vi "PathPlanner_Trajectory_Sample.vi"(9 "Time":dbl, 11 "PathPlannerTrajectory":T6 {"States"."HolonomicRotation"."SIN" format="%13.4f"; "States"."HolonomicRotation"."COS" format="%13.4f"; "States"."HolonomicRotation"."VALUE" format="%13.4f"; "States"."AngularVelocity"."SIN" format="%13.4f"; "States"."AngularVelocity"."COS" format="%13.4f"; "States"."AngularVelocity"."VALUE" format="%13.4f"; "States"."TrajectoryState"."POSE"."ROTATION"."SIN" format="%13.4f"; "States"."TrajectoryState"."POSE"."ROTATION"."COS" format="%13.4f"; "States"."TrajectoryState"."POSE"."ROTATION"."VALUE" format="%13.4f"; "States"."TrajectoryState"."POSE"."TRANSLATION"."Y" format="%14.3f"; "States"."TrajectoryState"."POSE"."TRANSLATION"."X" format="%14.3f"; "States"."AngularAcceleration"."SIN" format="%13.4f"; "States"."AngularAcceleration"."COS" format="%13.4f"; "States"."AngularAcceleration"."VALUE" format="%13.4f"}) -> (3 "PathPlannerState":T1={"AngularAcceleration"={"VALUE"=0.0, "COS"=1.0, "SIN"=0.0}, "PositionMeters"=0.0, "TrajectoryState"={"TimeSeconds"=0.0, "Velocity"=0.0, "Acceleration"=0.0, "POSE"={"TRANSLATION"={"X"=0.0, "Y"=0.0}, "ROTATION"={"VALUE"=0.0, "COS"=1.0, "SIN"=0.0}}, "Curvature"=0.0}, "AngularVelocity"={"VALUE"=0.0, "COS"=1.0, "SIN"=0.0}, "HolonomicRotation"={"VALUE"=0.0, "COS"=1.0, "SIN"=0.0}, "CurveRadius"=0.0, "DeltaPos"=0.0} {"HolonomicRotation"."SIN" format="%13.4f"; "HolonomicRotation"."COS" format="%13.4f"; "HolonomicRotation"."VALUE" format="%13.4f"; "AngularVelocity"."SIN" format="%13.4f"; "AngularVelocity"."COS" format="%13.4f"; "AngularVelocity"."VALUE" format="%13.4f"; "TrajectoryState"."POSE"."ROTATION"."SIN" format="%13.4f"; "TrajectoryState"."POSE"."ROTATION"."COS" format="%13.4f"; "TrajectoryState"."POSE"."ROTATION"."VALUE" format="%13.4f"; "TrajectoryState"."POSE"."TRANSLATION"."Y" format="%14.3f"; "TrajectoryState"."POSE"."TRANSLATION"."X" format="%14.3f"; "AngularAcceleration"."SIN" format="%13.4f"; "AngularAcceleration"."COS" format="%13.4f"; "AngularAcceleration"."VALUE" format="%13.4f"})   [LabVIEW 2019, in "PathPlanner.lvlib"]
doc: "Sample the path at a point in time\n\nInputs:\n - time -- The time to sample\n\nOutputs:\n - PathPlannerState -- The state at the given point in time"
uses:
  PathPlanner.lvlib
  PathPlannerTrajectory.ctl
  PathPlannerState.ctl
  <vilib>/Rock Robotics/WPI/ThirdParty/JAS_Junk/TrajLib/ROTATION2D.ctl
  <vilib>/Rock Robotics/WPI/ThirdParty/JAS_Junk/TrajLib/TRAJ_STATE.ctl
  <vilib>/Rock Robotics/WPI/ThirdParty/JAS_Junk/TrajLib/POSE2D.ctl
  <vilib>/Rock Robotics/WPI/ThirdParty/JAS_Junk/TrajLib/TRANSLATION2D.ctl
  <vilib>/Rock Robotics/WPI/ThirdParty/JAS_Junk/TrajLib/Trajectory_Library.lvlib
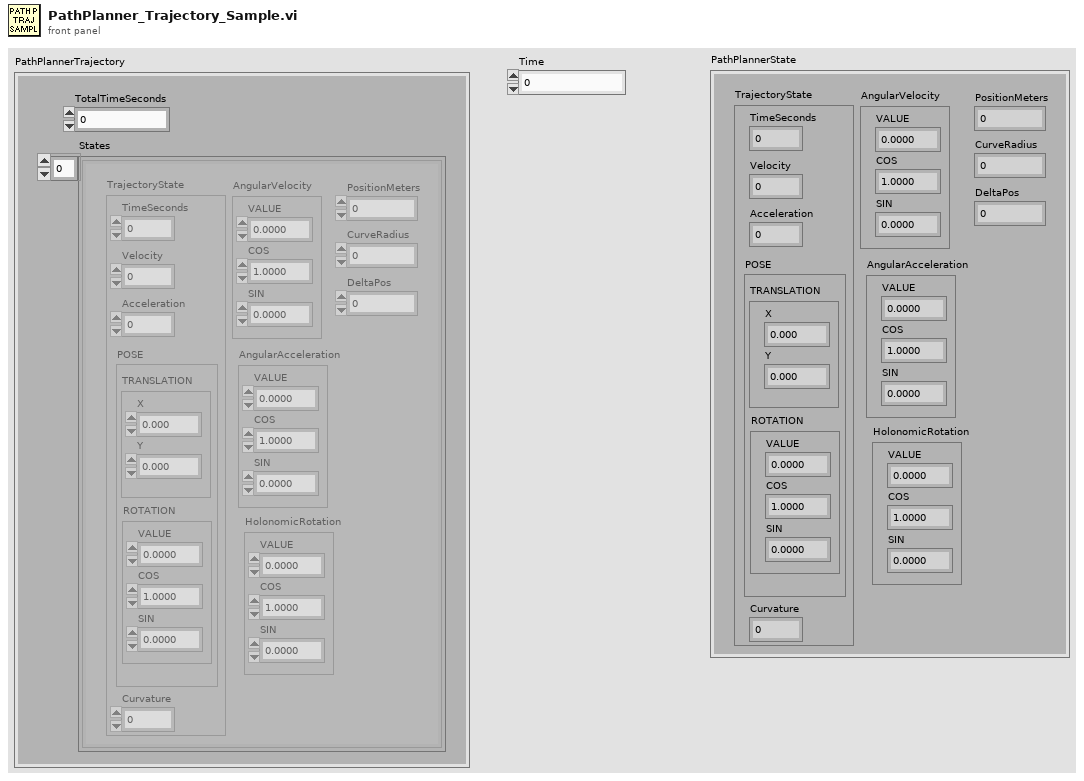
[diagram p1: front panel]
types:
  T1 = typedef "PathPlanner.lvlib/PathPlannerState.ctl" = cluster{"AngularAcceleration":T2, "PositionMeters":dbl, "TrajectoryState":T3, "AngularVelocity":T2, "HolonomicRotation":T2, "CurveRadius":dbl, "DeltaPos":dbl}
  T2 = typedef "Trajectory_Library.lvlib/ROTATION2D.ctl" = cluster{"VALUE":dbl, "COS":dbl, "SIN":dbl}
  T3 = typedef "Trajectory_Library.lvlib/TRAJ_STATE.ctl" = cluster{"TimeSeconds":dbl, "Velocity":dbl, "Acceleration":dbl, "POSE":T4, "Curvature":dbl}
  T4 = typedef "Trajectory_Library.lvlib/POSE2D.ctl" = cluster{"TRANSLATION":T5, "ROTATION":T2}
  T5 = typedef "Trajectory_Library.lvlib/TRANSLATION2D.ctl" = cluster{"X":dbl, "Y":dbl}
  T6 = typedef "PathPlanner.lvlib/PathPlannerTrajectory.ctl" = cluster{"TotalTimeSeconds":dbl, "States":T1[]}
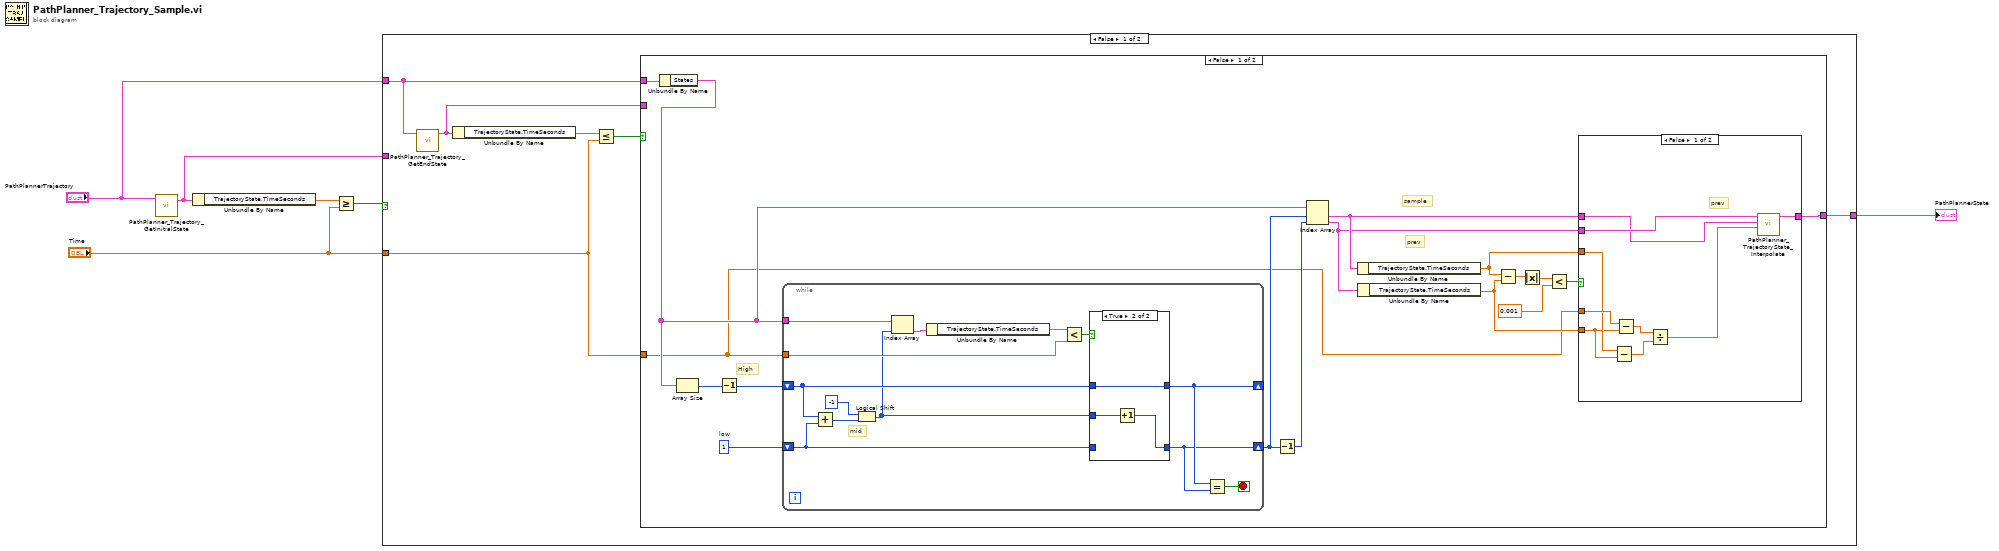
[diagram p0: block diagram]
diagram:
  n1 = call "PathPlanner_Trajectory_GetInitialState.vi"("PathPlannerTrajectory"="PathPlannerTrajectory") -> ("PathPlannerState"=w4:T1)  [unwired: 10 in]
  n2 = Unbundle By Name(w4) -> ("TrajectoryState.TimeSeconds"=w6:dbl)
  n3 = Greater Or Equal?(x=w6, y="Time") -> (x >= y?=w5:bool)
  n4 = case shown="False" w5 {
    tunnel: w4 -> [_ w59]
    tunnel: [w9 w59] -> w1
    tunnel: "PathPlannerTrajectory" -> [w8 _]
    tunnel: "Time" -> [w7 _]
    frame False {
      n5 = call "PathPlanner_Trajectory_GetEndState.vi"("PathPlannerTrajectory"=w8) -> ("PathPlannerState"=w10:T1)  [unwired: 10 in]
      n6 = Unbundle By Name(w10) -> ("TrajectoryState.TimeSeconds"=w12:dbl)
      n7 = Less Or Equal?(x=w12, y=w7) -> (x <= y?=w11:bool)
      n8 = case shown="False" w11 {
        tunnel: w10 -> [_ w58]
        tunnel: [w17 w58] -> w9
        tunnel: w8 -> [w29 _]
        tunnel: w7 -> [w14 _]
        frame False {
          w26 = 1  # low
          # "prev"
          # "sample"
          # "High"
          n9 = Unbundle By Name(w29) -> ("States"=w25:T1[])
          n10 = Array Size(array=w25) -> (size(s)=w28:i32)
          n11 = Decrement(x=w28) -> (x-1=w27:i32)
          n12 = while {
            shift-right: [w40] -> w24
            shift-left: w26 -> [w42]
            shift-right: [w41] -> _
            shift-left: w27 -> [w44]
            tunnel: w25 -> [w49]
            tunnel: w14 -> [w46]
            stop <- w50 stop-if-true
            # "mid"
            n13 = Add(x=w44, y=w42) -> (x+y=w52:i32)
            n14 = Logical Shift(y=i16 -1, x=w52) -> (x << y=w43:i32)
            n15 = Index Array(array=w49, index=w43) -> (element=w48:T1)
            n16 = Unbundle By Name(w48) -> ("TrajectoryState.TimeSeconds"=w47:dbl)
            n17 = Less?(x=w47, y=w46) -> (x < y?=w45:bool)
            n18 = case shown="True" w45 {
              tunnel: w44 -> [_ w57]
              tunnel: [w53 w57] -> w41
              tunnel: w43 -> [w53 w56]
              tunnel: w42 -> [w54 _]
              tunnel: [w54 w55] -> w40
              frame False {
              }
              frame True {
                n19 = Increment(x=w56) -> (x+1=w55:i32)
              }
            }
            n20 = Equal?(x=w41, y=w40) -> (x = y?=w50:bool)
          }
          n21 = Decrement(x=w24) -> (x-1=w23:i32)
          n22 = Index Array(array=w25, index #1=w24, index #2=w23) -> (element #1=w18:T1, element #2=w16:T1)
          n23 = Unbundle By Name(w18) -> ("TrajectoryState.TimeSeconds"=w13:dbl)
          n24 = Unbundle By Name(w16) -> ("TrajectoryState.TimeSeconds"=w15:dbl)
          n25 = Subtract(x=w13, y=w15) -> (x-y=w22:dbl)
          n26 = Absolute Value(x=w22) -> (abs(x)=w21:dbl)
          n27 = Less?(x=w21, y=0.001) -> (x < y?=w19:bool)
          n28 = case shown="False" w19 {
            tunnel: w18 -> [w31 w39]
            tunnel: [w38 w39] -> w17
            tunnel: w16 -> [w32 _]
            tunnel: w15 -> [w35 _]
            tunnel: w14 -> [w37 _]
            tunnel: w13 -> [w36 _]
            frame False {
              # "prev"
              n29 = Subtract(x=w36, y=w35) -> (x-y=w33:dbl)
              n30 = Subtract(x=w37, y=w35) -> (x-y=w34:dbl)
              n31 = Divide(x=w34, y=w33) -> (x/y=w30:dbl)
              n32 = call "PathPlanner_TrajectoryState_Interpolate.vi"("Time"=w30, "end Val"=w31, "in PathPlannerState"=w32) -> ("interpolated PathPlanner State"=w38:T1)  [unwired: 8 in]
            }
            frame True {
            }
          }
        }
        frame True {
        }
      }
    }
    frame True {
    }
  }
  "PathPlannerState" <- w1
